vi "Create Folders if Necessary.vi"(0 "Report Directory IN":path, 11 "Error IN":errorcluster) -> (4 "Report Directory OUT":path, 15 "Error OUT":errorcluster)   [LabVIEW 2011]
panel:
  out "Folders to Create":path[](array[path])
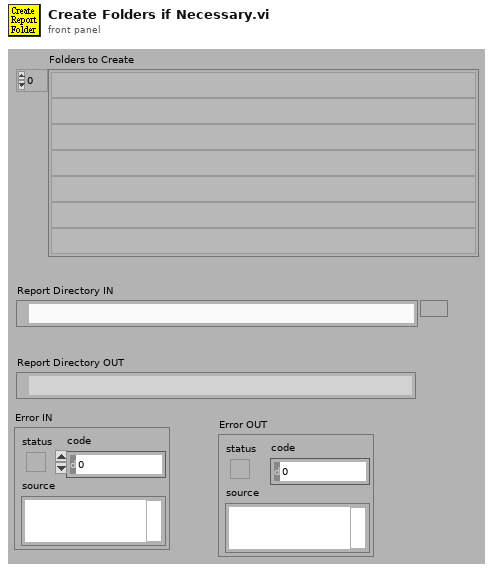
[diagram p1: front panel]
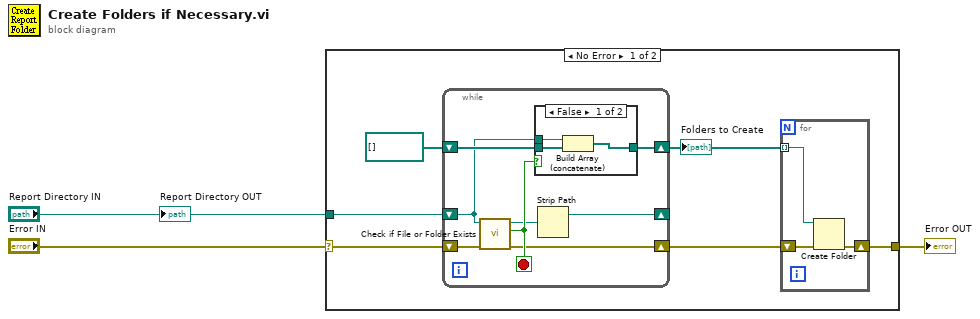
[diagram p0: block diagram]
diagram:
  n1 = case shown="No Error" "Error IN" {
    selector: "Error IN" -> [w4 w25]
    tunnel: "Report Directory IN" -> [w8 _]
    tunnel: [w5 w25] -> w3
    frame No Error {
      n2 = while {
        shift-right: [w17] -> _
        shift-left: w8 -> [w14]
        shift-right: [w19] -> w6
        shift-left: path[] [] -> [w20]
        shift-right: [w16] -> w7
        shift-left: w4 -> [w15]
        stop <- w18 stop-if-true
        n3 = call <vilib>:"Check if File or Folder Exists.vi"("error in (no error)"=w15, "path"=w14) -> ("error out"=w16:errorcluster, "file or folder exists?"=w18:bool, "dup path"=w13:path)  [unwired: 7 out]
        n4 = case shown="False" w18 {
          tunnel: w20 -> [w23 w24]
          tunnel: [w22 w24] -> w19
          tunnel: w14 -> [w21 _]
          frame False {
            n5 = Build Array (concatenate)(w21, w23) -> (w22:path[])
          }
          frame True {
          }
        }
        n6 = Strip Path(path=w13) -> (stripped path=w17:path)  [unwired: 1 out]
      }
      "Folders to Create" <- w6
      n7 = for {
        shift-right: [w11] -> w5
        shift-left: w7 -> [w12]
        tunnel: w6 -> [w10] mode=indexing
        n8 = Create Folder(path (use dialog)=w10, error in=w12) -> (error out=w11:errorcluster)  [unwired: 3 out]
      }
    }
    frame Error {
    }
  }
  "Error OUT" <- w3
  "Report Directory OUT" <- "Report Directory IN"
